vi "SVFA Get Waterfall Value (Array X).vi"(0 "waterfall data":T1, 2 "x values":dbl[](array[numeric]), 3 "coercion (nearest)":T8(ring), 4 "spectrum info":T2 {"x-axis units" items=["Time (s)"=0, "Frequency-CB (Hz)"=1, "Frequency-CPB (Hz)"=1248, "Frequency-Arbitrary (Hz)"=2357, "Quefrency (s)"=2, "Revolutions (rev)"=3, "Order"=4, "Speed (RPM)"=11, "Speed (rad/s)"=21, "Index"=65535]; "weighting filter" items=["Linear", "A-weighting", "B-weighting", "C-weighting", "ITU-R 468-4", "Dolby", "CCITT", "C-message", "Wb", "Wc", "Wd", "We", "Wf", "Wh", "Wj", "Wk", "Wm", "AES17 20 kHz lowpass", "AES17 40 kHz lowpass", "AES17 20 kHz highpass", "AES17 40 kHz highpass"]; "dB reference [EU]" format="%.2f"; "engineering units" items=["custom..."=0, "V"=1, "A"=21, "C"=30, "pC"=31, "s"=32, "-"=29, "Pa"=2, "N"=20, "g"=3, "m/s^2"=4, "m/s"=5, "m"=6, "mm/s"=12, "mm"=13, "micron/s"=14, "micron"=15, "in/s^2"=7, "in/s"=8, "in"=9, "mil/s"=10, "mil"=11, "rad/s^2"=16, "rad/s"=17, "rad"=18, "deg/s^2"=26, "deg/s"=27, "deg"=28, "RPM"=22, "cycle/s^2"=23, "Hz"=24, "cycle"=25, "strain"=19]; "spectral info"."window" items=["None "=0, "Hanning"=1, "Hamming"=2, "Blackman-Harris"=3, "Exact Blackman"=4, "Blackman"=5, "Flat Top"=6, "4 Term B-Harris "=7, "7 Term B-Harris"=8, "Low Sidelobe"=9, "Force - Exponential"=10, "Gaussian"=62]}, 5 "error in":errorcluster) -> (14 "waterfall values":cluster{"X":dbl, "Y":dbl, "Z":dbl}[](array[cluster]), 19 "error out":errorcluster)   [LabVIEW 2017]
doc: "Extracts the value of the spectrum at the specified frequency. Use the frequency coercion control to specify how the frequency should be coerced if it does not exactly coincide with a frequency line. This VI operates on any real-valued spectrum. Wire data to the <B>spectrum</B> input to determine the polymorphic instance to use or manually select the instance."
uses:
  <vilib>/addons/_NISVFA/_Shared subVIs/Controls/svc_Spectrum Info.ctl
  <vilib>/addons/_NISVFA/_Shared subVIs/Controls/svc_X-Axis Units.ctl
  <vilib>/addons/_NISVFA/_Shared subVIs/Controls/svc_Spectrum Type.ctl
  <vilib>/addons/_NISVFA/_Shared subVIs/Controls/svc_Engineering Units Text Ring.ctl
  <vilib>/addons/_NISVFA/_Shared subVIs/Controls/svc_Weighting Filter Text Ring.ctl
  <vilib>/addons/_NISVFA/_Shared subVIs/Controls/svc_Complimentary Spectrum Units.ctl
  <vilib>/addons/_NISVFA/_Spectrum Processing/SVFA Get Spectrum Value (1 Ch).vi
  <vilib>/addons/_NISVFA/_Shared subVIs/Common/svc_Spectrum Units.vi
  <vilib>/addons/_NISVFA/_Shared subVIs/Common/svc_Convert Frequency to Frequency String.vi
  <vilib>/addons/_NISVFA/_Shared subVIs/Common/svc_Get Weighting Enum and Labels.vi
  <vilib>/addons/_NISVFA/_Shared subVIs/Common/svc_Unit Label Lexical Class.vi
  <vilib>/addons/_NISVFA/_Shared subVIs/Common/svc_Engineering Units to Unit Label.vi
  <vilib>/addons/_NISVFA/_Shared subVIs/Common/svc_Format Value (DBL).vi
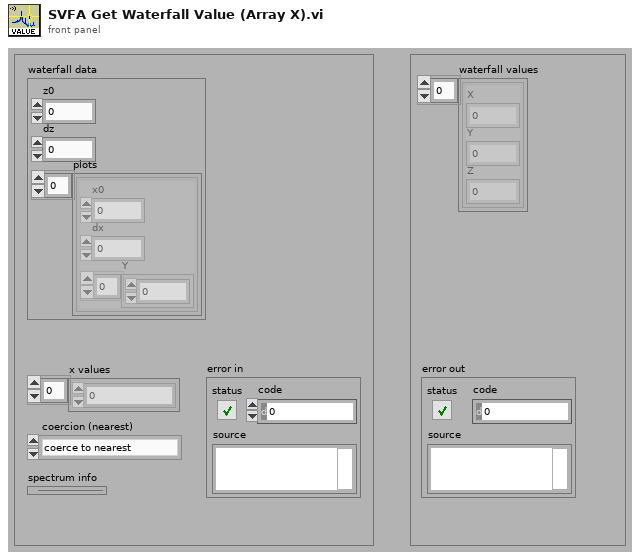
[diagram p1: front panel]
types:
  T1 = cluster{"z0":dbl, "dz":dbl, "plots":cluster{"x0":dbl, "dx":dbl, "Y":dbl[]}[]}
  T2 = typedef "svc_Spectrum Info.ctl" = cluster{"channel name":string, "description":string, "x-axis units":T3, "spectral info":cluster{"spectrum type":T4, "linear/dB":enum16{"linear", "dB"}, "window":u16, "window size":i32, "FFT size":i32}, "engineering units":T5, "custom label":string, "dB reference [EU]":dbl, "peak units":enum16{"rms", "peak", "peak-peak"}, "weighting filter":T6, "spectral density?":bool, "unit label":string, "spectrum skewed?":bool, "complimentary spectrum units":T7}
  T3 = typedef "svc_X-Axis Units.ctl" = u16
  T4 = typedef "svc_Spectrum Type.ctl" = enum16{"FFT Spectrum [complex]", "Amplitude [Magnitude]", "Power [Magnitude^2]", "Cross Spectrum [complex]", "Frequency Response [Complex]"}
  T5 = typedef "svc_Engineering Units Text Ring.ctl" = u16
  T6 = typedef "svc_Weighting Filter Text Ring.ctl" = u16
  T7 = typedef "svc_Complimentary Spectrum Units.ctl" = enum16{"none", "radians", "degrees", "cycles", "imaginary"}
  T8 = enum16{"coerce to nearest", "coerce to next highest", "coerce to next lowest", "interpolate"}
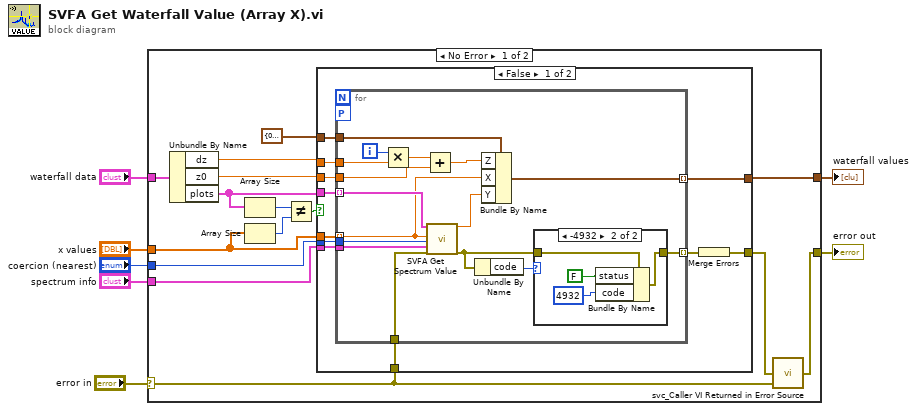
[diagram p0: block diagram]
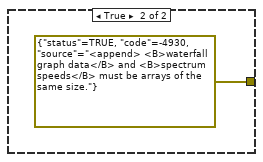
[diagram p3: hidden frame]
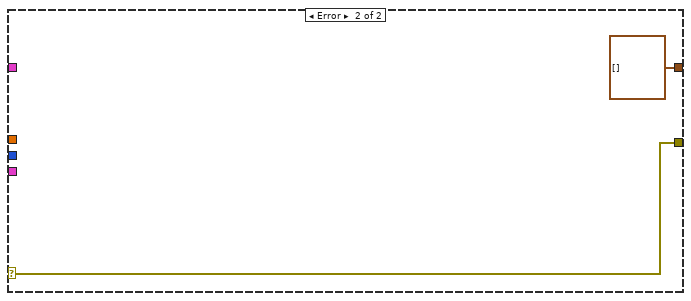
[diagram p4: hidden frame]
diagram:
  n1 = case shown="No Error" "error in" {
    selector: "error in" -> [w8 w57]
    tunnel: [w9 w57] -> w7
    tunnel: "x values" -> [w19 _]
    tunnel: "coercion (nearest)" -> [w18 _]
    tunnel: [w17 cluster{"X":dbl, "Y":dbl, "Z":dbl}[] []] -> w4
    tunnel: "spectrum info" -> [w16 _]
    tunnel: "waterfall data" -> [w14 _]
    frame No Error {
      n2 = Unbundle By Name(w14) -> ("dz"=w13:dbl, "z0"=w12:dbl, "plots"=w11:cluster{"x0":dbl, "dx":dbl, "Y":dbl[]}[])
      n3 = Array Size(array=w11) -> (size(s)=w20:i32)
      n4 = Array Size(array=w19) -> (size(s)=w21:i32)
      n5 = Not Equal?(x=w20, y=w21) -> (x != y?=w22:bool)
      n6 = case shown="False" w22 {
        tunnel: cluster{"X":dbl, "Y":dbl, "Z":dbl} {"X"=0.0, "Y"=0.0, "Z"=0.0} -> [w33 _]
        tunnel: w16 -> [w32 _]
        tunnel: [w28 _] -> w17
        tunnel: w18 -> [w31 _]
        tunnel: w11 -> [w30 _]
        tunnel: w19 -> [w29 _]
        tunnel: [w25 errorcluster {"status"=TRUE, "code"=-4930, "source"="<append> <B>waterfall graph data</B> and <B>spectrum speeds</B> must be arrays of the same size."} ("error in")] -> w10
        tunnel: w13 -> [w27 _]
        tunnel: w12 -> [w26 _]
        tunnel: w8 -> [w23 _]
        frame False {
          n7 = for {
            tunnel: w30 -> [w49] mode=indexing
            tunnel: w33 -> [w48]
            tunnel: [w47] -> w28 mode=indexing
            tunnel: w32 -> [w45]
            tunnel: w29 -> [w35] mode=indexing
            tunnel: w31 -> [w44]
            tunnel: w27 -> [w42]
            tunnel: w26 -> [w40]
            workers-P: _ -> [_]
            tunnel: [w36] -> w24 mode=indexing
            tunnel: w23 -> [w34]
            i -> [w43]
            n8 = Multiply(x=w43, y=w42) -> (x*y=w41:dbl)
            n9 = Add(x=w41, y=w40) -> (x+y=w39:dbl)
            n10 = call-poly <vilib>:"SVFA Get Spectrum Value.vi"("spectrum"=w49, "x value (1000)"=w35, "coercion (nearest)"=w44, "spectrum info"=w45, "error in (no error)"=w34) -> ("spectrum value"=w46:dbl, "error out"=w37:errorcluster)  [unwired: 10 in, 3 out]
            n11 = Unbundle By Name(w37) -> ("code"=w38:i32)
            n12 = Bundle By Name(cluster=w48, "Z"=w39, "X"=w35, "Y"=w46) -> (w47:cluster{"X":dbl, "Y":dbl, "Z":dbl})
            n13 = case shown="-4932" w38 {
              tunnel: [w50 w52] -> w36
              tunnel: w37 -> [w50 w51]
              frame Default {
              }
              frame -4932 {
                n14 = Bundle By Name(cluster=w51, "status"=FALSE, "code"=4932) -> (w52:errorcluster)
              }
            }
          }
          n15 = Merge Errors(w24) -> (w25:errorcluster)
        }
        frame True {
        }
      }
      n16 = call <vilib>:"svc_Caller VI Returned in Error Source.vi"("warning input to caller"=w8, "error in (no error)"=w10) -> ("error out"=w9:errorcluster)  [unwired: 3 in]
    }
    frame Error {
    }
  }
  "error out" <- w7
  "waterfall values" <- w4
